vi "Refresh_AScan (SubVI).vi"(8 "error in":errorcluster, 11 "WaveformGraph in":refnum<vi>) -> (0 "error out":errorcluster)   [LabVIEW 2017]
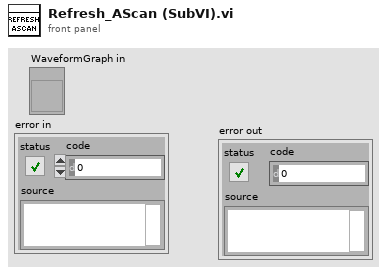
[diagram p1: front panel]
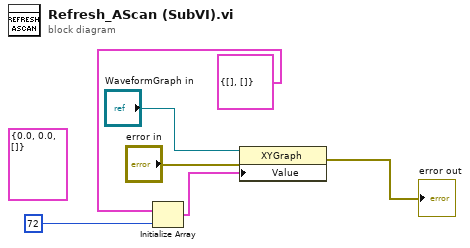
[diagram p0: block diagram]
diagram:
  (unwired) cluster{"f0":dbl, "df":dbl, "magnitude":dbl[]} {"f0"=0.0, "df"=0.0, "magnitude"=[]} ("magnitude")
  n1 = Initialize Array(cluster{dbl[], dbl[]} {[], []} ("XY Graph"), 72 ("dimension size")) -> (w6:cluster{dbl[], dbl[]}[])
  n2 = property class="XYGraph"(reference="WaveformGraph in", error in="error in", "Value"=w6) -> (error out=→"error out":errorcluster)  [unwired: 1 out]
